vi "Draw Circle.vi"(10 "r":dbl, 11 "Center":cluster{"x":dbl, "y":dbl} {"y" scale=-10.0..10.0; "x" scale=-10.0..10.0}) -> (3 "circle":cluster{dbl[], dbl[]})   [LabVIEW 2019, in "Pure Pursuit.lvlib"]
uses:
  Pure Pursuit.lvlib
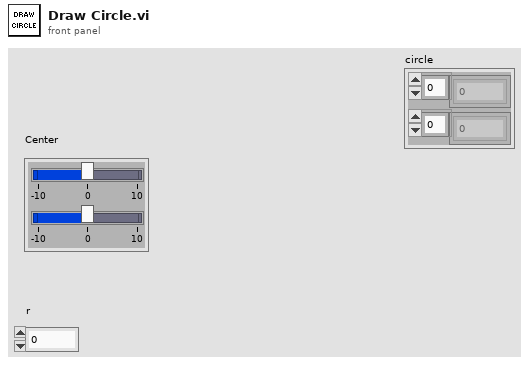
[diagram p1: front panel]
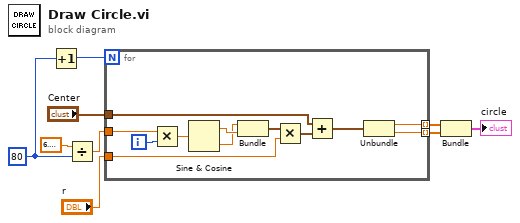
[diagram p0: block diagram]
diagram:
  w4 = 80
  n1 = Increment(x=w4) -> (x+1=w5:i32)
  n2 = Divide(x=6.283185307179586, y=w4) -> (x/y=w7:dbl)
  n3 = for {
    N: w5 -> [_]
    tunnel: "Center" -> [w14]
    tunnel: w7 -> [w21]
    tunnel: "r" -> [w15]
    tunnel: [w11] -> w3 mode=indexing
    tunnel: [w10] -> w2 mode=indexing
    i -> [w20]
    n4 = Multiply(x=w21, y=w20) -> (x*y=w19:dbl)
    n5 = Sine & Cosine(0:w19) -> (1:w18:dbl, 2:w17:dbl)
    n6 = Bundle(w17, w18) -> (w16:cluster{dbl, dbl})  [unwired: 1 in]
    n7 = Multiply(x=w16, y=w15) -> (x*y=w13:cluster{dbl, dbl})
    n8 = Add(x=w14, y=w13) -> (x+y=w12:cluster{dbl, dbl})
    n9 = Unbundle(w12) -> (w11:dbl, w10:dbl)
  }
  n10 = Bundle(w3, w2) -> (→"circle":cluster{dbl[], dbl[]})  [unwired: 1 in]
